vi "Read Data Model.vi"(8 "error in (no error)":errorcluster, 11 "Modbus slave in":refnum<class "Modbus Master CR API.lvclass">) -> (0 "error out":errorcluster, 2 "device data model":refnum<class "Device Data Model.lvclass">, 3 "Modbus slave out":refnum<class "Modbus Master CR API.lvclass">)   [LabVIEW 2021, in "Modbus Master CR API.lvclass"]
doc: "This VI is an accessor for the <B>data model</B> stored in the Modbus master instance. This accessor can be used as a property node. This model defines how the slave stores data and reacts to functions and data sent by a Modbus master."
uses:
  Modbus Master CR API.lvclass
  D:/my_projects/projects/Algorithms/Labview/21/Modbus_v121c/API/Modbus API.lvclass
  Data Model/Device Data Model.lvclass
  Modbus API.lvclass/Modbus API.ctl
  Modbus Master CR API.lvclass/Modbus Master CR API.ctl
  Network Protocol/MB/Modbus Master CR.lvclass
  Modbus API.lvclass
  D:/my_projects/projects/Algorithms/Labview/21/Modbus_v121c/API/Modbus Master CR API/Modbus Master CR API.lvclass
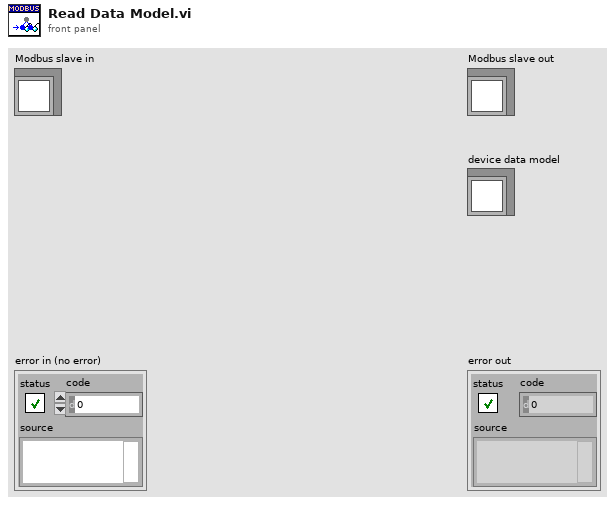
[diagram p1: front panel]
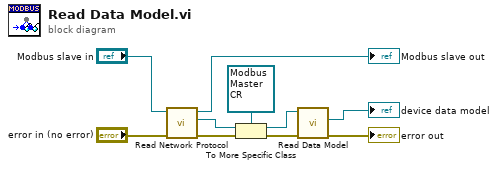
[diagram p0: block diagram]
diagram:
  n1 = call "Read Network Protocol.vi"("error in (no error)"="error in (no error)", "Modbus API in"="Modbus slave in") -> ("error out"=w8:errorcluster, "Network Protocol"=w9:refnum<class "Network Protocol.lvclass">, "Modbus API out"=→"Modbus slave out":refnum<class "Modbus Master CR API.lvclass">)  [unwired: 7 in]
  n2 = To More Specific Class(target class=refnum<class "Modbus Master CR.lvclass"> refnum ("Modbus Master CR.lvclass"), reference=w9, error in=w8) -> (specific class reference=w1:refnum<class "Modbus Master CR.lvclass">, error out=w4:errorcluster)
  n3 = call "Read Data Model.vi"("error in (no error)"=w4, "MB_TCP in"=w1) -> ("error out"=→"error out":errorcluster, "Data Model"=→"device data model":refnum<class "Device Data Model.lvclass">)  [unwired: 7 in, 1 out]
